vi "set_clock_enabled_state.vi"(8 "error in (no error)":errorcluster, 10 "enable clocks?":bool, 11 "FPGAWrapperAN110607Galvo in":refnum<class "FPGAWrapperAN110607Galvo.lvclass">) -> (0 "error out":errorcluster, 3 "FPGAWrapperAN110607Galvo out":refnum<class "FPGAWrapperAN110607Galvo.lvclass">)   [LabVIEW 2010, in "FPGAWrapperAN110607Galvo.lvclass"]
uses:
  FPGAWrapperAN110607Galvo.lvclass
  GenericFPGAWrapper/GenericFPGAWrapper/GenericFPGAWrapper.lvclass
  <vilib>/rvi/interface/nirviReadWriteControl/nirviReadWriteControl.xnode
  FPGA_VI_ref.ctl
  <vilib>/rvi/interface/common/niFpgaNodeNameForErrorReporting.ctl
  <vilib>/rvi/errors/niLvFpgaWhatHappensToTopLevelVI.ctl
  <vilib>/Utility/error.llb/Error Cluster From Error Code.vi
  <vilib>/rvi/errors/niLvFpgaAdjustHostInterfaceError.vi
  NiFpgaLv.dll
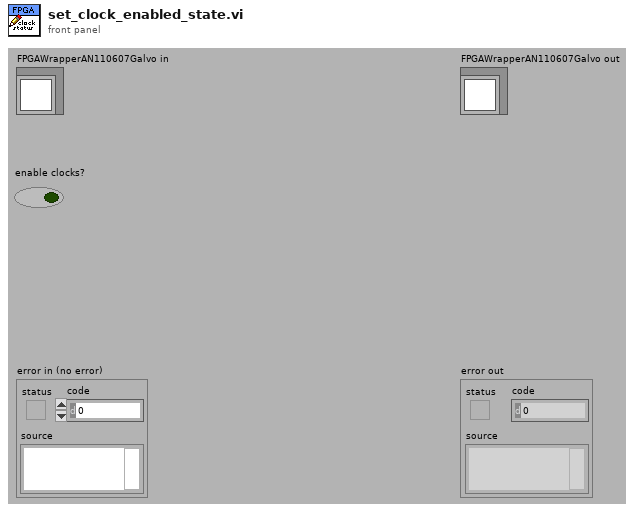
[diagram p1: front panel]
types:
  T1 = typedef "niFpgaNodeNameForErrorReporting.ctl" = enum16{"Open FPGA VI Reference", "Read/Write Control", "Invoke Method: Abort", "Invoke Method: Acknowledge IRQ", "Invoke Method: Download", "Invoke Method: FIFO.Configure", "Invoke Method: FIFO.Read", "Invoke Method: FIFO.Start", "Invoke Method: FIFO.Stop", "Invoke Method: FIFO.Write", "Invoke Method: Reset", "Invoke Method: Run", "Invoke Method: Wait on IRQ", "Close FPGA VI Reference"}
  T2 = typedef "niLvFpgaWhatHappensToTopLevelVI.ctl" = enum16{"top level VI scripted behind XNode", "top level VI inlined behind XNode"}
  T3 = typedef "FPGAWrapperAN110607Galvo.lvclass/FPGA_VI_ref.ctl" = refnum<k20>
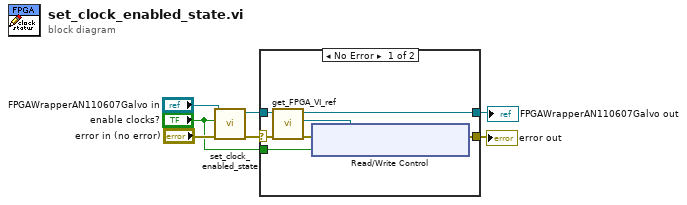
[diagram p0: block diagram]
diagram:
  n1 = call-parent "set_clock_enabled_state.vi"("error in (no error)"="error in (no error)", "enable clocks?"="enable clocks?", "GenericFPGAWrapper in"="FPGAWrapperAN110607Galvo in") -> ("error out"=w4:errorcluster, "GenericFPGAWrapper out"=w5:refnum<class "FPGAWrapperAN110607Galvo.lvclass">)  [unwired: 7 in]
  n2 = case shown="No Error" w4 {
    selector: w4 -> [w11 w54]
    tunnel: w5 -> [w14 w55]
    tunnel: [w10 w54] -> w3
    tunnel: [w9 w55] -> w2
    tunnel: "enable clocks?" -> [w8 _]
    frame No Error {
      n3 = call-dynamic "get_FPGA_VI_ref.vi"("error in (no error)"=w11, "FPGAWrapperAN110607Galvo in"=w14) -> ("error out"=w13:errorcluster, "FPGA VI reference"=w12:T3, "FPGAWrapperAN110607Galvo out"=w9:refnum<class "FPGAWrapperAN110607Galvo.lvclass">)  [unwired: 7 in]
      n4 = xnode "Read/Write Control"("FPGA VI Reference In"=w12, "error in"=w13, "shall  acquisition start clocks?"=w8) -> ("error out"=w10:errorcluster)  [unwired: 1 out]
    }
    frame Error {
    }
  }
  "error out" <- w3
  "FPGAWrapperAN110607Galvo out" <- w2
